vi "testDifferent.vi"() -> (0 "error out":errorcluster)   [LabVIEW 2017, in "AssertionTest.lvlib" / "AssertEquals.lvlib"]
uses:
  AssertEquals.lvlib
  Assertion/Assertion.lvlib
  2789387b-9fc4-48d4-8fe2-4901f87429e4.vi
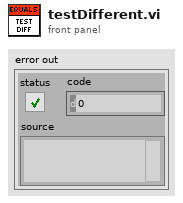
[diagram p1: front panel]
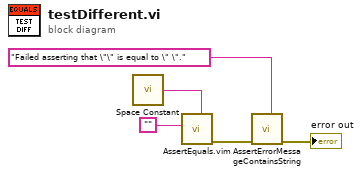
[diagram p0: block diagram]
diagram:
  n1 = call <vilib>:"Space Constant.vi"() -> ("String"=w4:string)
  n2 = call "AssertEquals.vim"("Expected"=w4, "Actual"="") -> ("error out"=w3:errorcluster)  [unwired: 9 in]
  n3 = call "AssertErrorMessageContainsString.vi"("Expected"="Failed asserting that \"\" is equal to \" \"." ("y"), "error in (no error)"=w3) -> ("error out"=→"error out":errorcluster)  [unwired: 9 in]
